vi "Calibration Mode.vi"(8 "error in (no error)":errorcluster, 10 "Enable":bool, 11 "ENET in":refnum<class "ENET_BS1201.lvclass">) -> (0 "error out":errorcluster, 3 "ENET out":refnum<class "ENET_BS1201.lvclass">)   [LabVIEW 2021, in "BS120x Driver.lvlib" / "ENET_BS1201.lvclass"]
doc: "Calibration mode disables the current calibration, removes all scaling, and returns bit counts."
uses:
  ENET_BS1201.lvclass
  C:/Users/Public/Documents/Projects/7100-00109 SW BS1201 LV Driver/trunk/source/ENET_BS120x/ENET_BS120x.lvclass
  ENET_BS120x/ENET_BS120x.lvclass
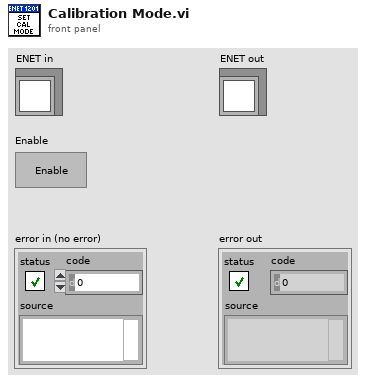
[diagram p1: front panel]
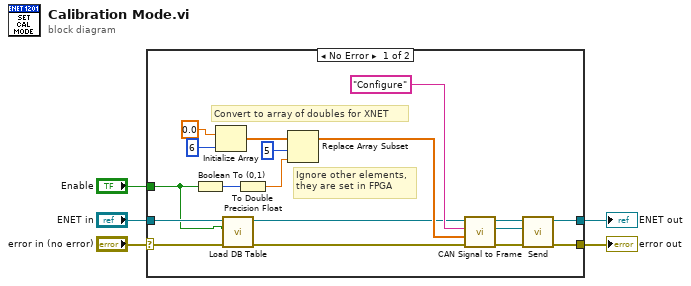
[diagram p0: block diagram]
diagram:
  n1 = case shown="No Error" "error in (no error)" {
    selector: "error in (no error)" -> [w9 w25]
    tunnel: [w12 w25] -> w4
    tunnel: [w13 w24] -> w2
    tunnel: "ENET in" -> [w10 w24]
    tunnel: "Enable" -> [w8 _]
    frame No Error {
      # "Ignore other elements,\nthey are set in FPGA"
      # "Convert to array of doubles for XNET"
      n2 = Boolean To (0,1)(Boolean=w8) -> (0, 1=w18:i16)
      n3 = Initialize Array(0.0 ("element"), 6 ("dimension size")) -> (w22:dbl[])
      n4 = call-dynamic "Load DB Table.vi"("error in (no error)"=w9, "Calibration Mode"=w8, "ENET in"=w10) -> ("error out"=w6:errorcluster, "ENET out"=w7:refnum<class "ENET_BS1201.lvclass">)  [unwired: 7 in]
      n5 = To Double Precision Float(number=w18) -> (double precision float=w23:dbl)
      n6 = Replace Array Subset(array=w22, new element=w23, index=5) -> (w17:dbl[])
      n7 = call "CAN Signal to Frame.vi"("error in (no error)"=w6, "Data Array"=w17, "Frame"="Configure", "ENET in"=w7) -> ("error out"=w11:errorcluster, "Data"=w14:refnum<class "Data.lvclass">, "ENET out"=w15:refnum<class "ENET_BS1201.lvclass">)  [unwired: 5 in]
      n8 = call "Send.vi"("error in (no error)"=w11, "Data"=w14, "ENET in"=w15) -> ("error out"=w12:errorcluster, "ENET out"=w13:refnum<class "ENET_BS1201.lvclass">)  [unwired: 7 in]
    }
    frame Error {
    }
  }
  "error out" <- w4
  "ENET out" <- w2
